vi "Running Event Handler.vi"(8 "error in (no error)":errorcluster, 10 "SessComplEvent":T1, 11 "Stim Player Data In":T2) -> (0 "error out":errorcluster, 2 "SessComplEvent dup":T1, 3 "Stim Player Data Out":T2, 4 "AllStimStopped?":bool)   [LabVIEW 2011]
uses:
  Controls/Stim Player Data.ctl
  Controls/Top Level Control.ctl
  <vilib>/NI/AMC/Message Queue.ctl
  <vilib>/NI/AMC/Message.ctl
  <vilib>/NI/Tools/Keyed Array/KeyedArray.ctl
  Controls/ListBox Test Record.ctl
  Controls/DVR of CSV Tests Data.ctl
  Controls/CSVs Tests Data.ctl
  Controls/Test Column Data.ctl
  Controls/Options DVR.ctl
  Controls/Options.ctl
  <vilib>/NI Veristand/Execution/Workspace/WorkspaceAPI.ctl
  NationalInstruments.VeriStand.ClientAPI
  <vilib>/NI Veristand/Execution/SequenceExecutionInterface/Stimulus Profile Session Ref.ctl
  <vilib>/NI Veristand/Execution/ChannelFaultManager/ChannelFaultAPI.ctl
  <vilib>/NI Veristand/Execution/SequenceExecutionInterface/Session Event Ref.ctl
  <vilib>/NI/AMC/Send Local Message.vi
  <vilib>/NI/AMC/Read Next Message.vi
  <vilib>/NI/AMC/Create Single Message.vi
  <vilib>/NI/AMC/Update Message Routing Info.vi
  <vilib>/NI/AMC/Read Termination Message.vi
  <vilib>/NI/AMC/Globals.vi
  <vilib>/NI Veristand/Execution/SequenceExecutionInterface/Stop Stimulus Profile Session.vi
  <vilib>/NI/AMC/Send Message.vi
  <vilib>/NI/Tools/Keyed Array/Tools_KeyedArray.lvlib
  <vilib>/NI/AMC/AMC.lvlib
  <vilib>/NI Veristand/Execution/Workspace/NI_VS Workspace ExecutionAPI.lvlib
  <vilib>/NI Veristand/Execution/SequenceExecutionInterface/NI_VS Sequence Execution Interface.lvlib
  <vilib>/NI Veristand/Execution/ChannelFaultManager/NI_VS ChannelFault ExecutionAPI.lvlib
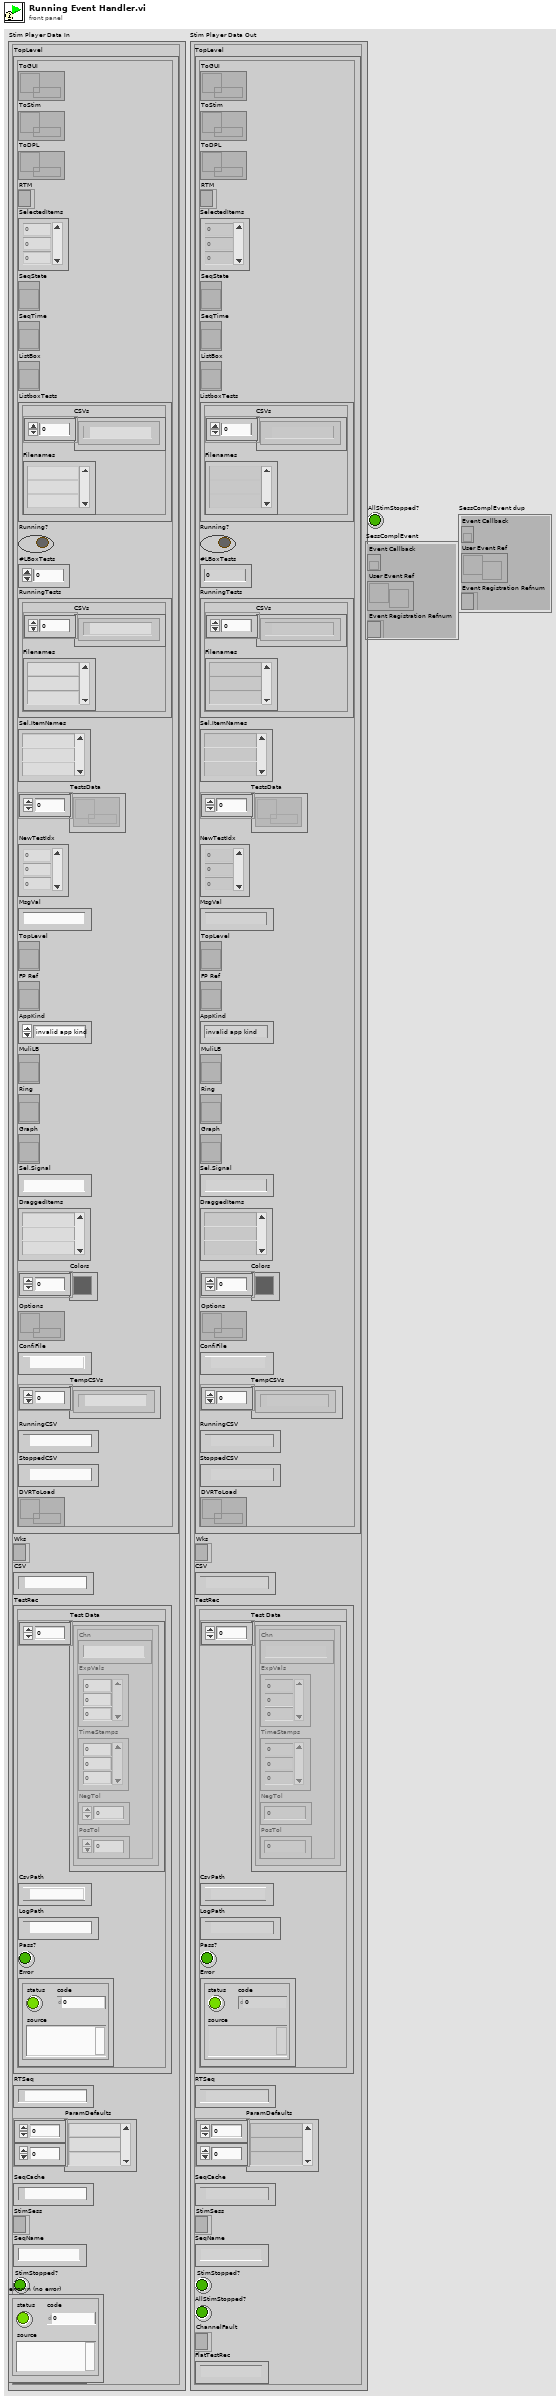
[diagram p1: front panel]
types:
  T1 = typedef "NI_VS Sequence Execution Interface.lvlib/Session Event Ref.ctl" = cluster{"Event Callback":refnum<k27>, "User Event Ref":refnum<user-event>, "Event Registration Refnum":refnum<event-registration>}
  T2 = typedef "Stim Player Data.ctl" = cluster{"TopLevel":T3, "Wks":T8, "CSV":path, "TestRec":T9, "RTSeq":path, "ParamDefaults":string[][], "SeqCache":path, "StimSess":T11, "SeqName":string, "StimStopped?":bool, "AllStimStopped?":bool, "ChannelFault":T12, "FlatTestRec":string}
  T3 = typedef "Top Level Control.ctl" = cluster{"ToGUI":T4, "ToStim":T4, "ToDPL":T4, "RTM":refnum<k9>, "SelectedItems":i32[], "SeqState":refnum<vi>, "SeqTime":refnum<vi>, "ListBox":refnum<vi>, "ListboxTests":T5, "Running?":bool, "#LBoxTests":i32, "RunningTests":T5, "Sel.ItemNames":string[], "TestsData":T6[], "NewTestIdx":i32[], "MsgVal":string, "TopLevel":refnum<vi>, "FP Ref":refnum<vi>, "AppKind":enum32{"invalid app kind", "Development System", "Run Time System", "Student Edition", "Embedded LabVIEW", "Evaluation", "Custom"}, "MuliLB":refnum<vi>, "Ring":refnum<vi>, "Graph":refnum<vi>, "Sel.Signal":string, "DraggedItems":string[], "Colors":u32[], "Options":T7, "ConfiFile":path, "TempCSVs":path[], "RunningCSV":path, "StoppedCSV":path, "DVRToLoad":T6}
  T4 = typedef "AMC.lvlib/Message Queue.ctl" = refnum<queue>
  T5 = typedef "ListBox Test Record.ctl" = cluster{"CSVs":path[], "Filenames":string[]}
  T6 = typedef "DVR of CSV Tests Data.ctl" = refnum<data-value>
  T7 = typedef "Options DVR.ctl" = refnum<data-value>
  T8 = typedef "NI_VS Workspace ExecutionAPI.lvlib/WorkspaceAPI.ctl" = refnum<k24>
  T9 = typedef "CSVs Tests Data.ctl" = cluster{"Test Data":T10[], "CsvPath":path, "LogPath":path, "Pass?":bool, "Error":errorcluster}
  T10 = typedef "Test Column Data.ctl" = cluster{"Chn":string, "ExpVals":dbl[], "TimeStamps":i64[], "NegTol":dbl, "PosTol":dbl}
  T11 = typedef "NI_VS Sequence Execution Interface.lvlib/Stimulus Profile Session Ref.ctl" = refnum<k24>
  T12 = typedef "NI_VS ChannelFault ExecutionAPI.lvlib/ChannelFaultAPI.ctl" = refnum<k24>
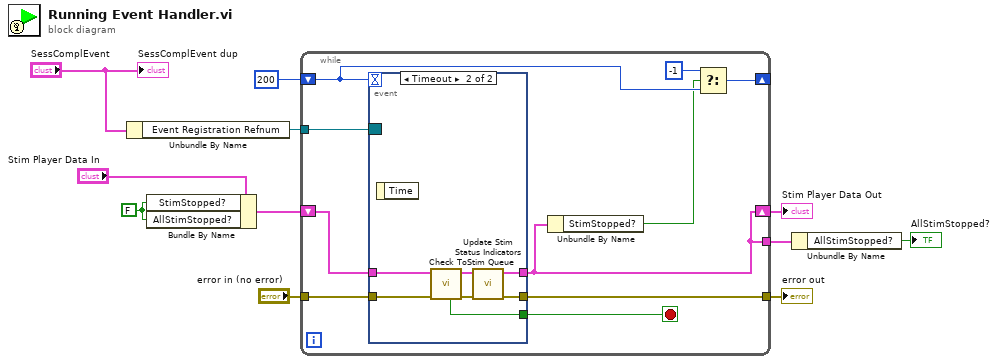
[diagram p0: block diagram]
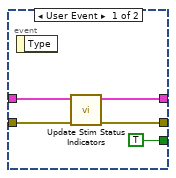
[diagram p2: hidden frame]
diagram:
  w8 = FALSE
  n1 = Unbundle By Name("SessComplEvent") -> ("Event Registration Refnum"=w5:refnum<event-registration>)
  n2 = Bundle By Name(cluster="Stim Player Data In", "StimStopped?"=w8, "AllStimStopped?"=w8) -> (w9:T2)
  n3 = while {
    tunnel: [w21] -> w11
    tunnel: "error in (no error)" -> [w19]
    shift-right: [w16] -> w7
    shift-left: w9 -> [w18]
    tunnel: w5 -> [w17]
    tunnel: [w16] -> w4
    shift-right: [w14] -> _
    shift-left: 200 -> [w15]
    stop <- w20 stop-if-true
    n4 = event shown="[1] Timeout" {
      selector: w17 -> [_ _]
      dyn-events: _ -> [_ _]
      timeout: w15 -> [_ _]
      tunnel: [w24 w32] -> w21
      tunnel: [TRUE w28] -> w20
      tunnel: w19 -> [w25 w31]
      tunnel: [w22 w33] -> w16
      tunnel: w18 -> [w23 w29]
      event User Event {
        n5 = event-data() -> ()  [unwired: 1 in, 1 out]
        n6 = call "Update Stim Status Indicators.vi"("error in (no error)"=w25, "Stim Player Data In"=w23) -> ("error out"=w24:errorcluster, "Stim Player Data Out"=w22:T2)  [unwired: 8 in]
      }
      event Timeout {
        n7 = event-data() -> ()  [unwired: 1 in, 1 out]
        n8 = call "Check ToStim Queue.vi"("error in (no error)"=w31, "Stim Player Data In"=w29) -> ("error out"=w30:errorcluster, "Stim Player Data Out"=w27:T2, "Error?"=w28:bool)  [unwired: 7 in]
        n9 = call "Update Stim Status Indicators.vi"("error in (no error)"=w30, "Stim Player Data In"=w27) -> ("error out"=w32:errorcluster, "Stim Player Data Out"=w33:T2)  [unwired: 8 in]
      }
    }
    n10 = Unbundle By Name(w16) -> ("StimStopped?"=w12:bool)
    n11 = Select(t=-1, s=w12, f=w15) -> (s? t:f=w14:i32)
  }
  "error out" <- w11
  "Stim Player Data Out" <- w7
  n12 = Unbundle By Name(w4) -> ("AllStimStopped?"=→"AllStimStopped?":bool)
  "SessComplEvent dup" <- "SessComplEvent"
